vi "Config FTPSync.vi"(8 "error in (no error)":errorcluster, 11 "Cluster":T1) -> (0 "error out":errorcluster, 3 "FTPProtocol out":refnum<class "FTPProtocol.lvclass">)   [LabVIEW 2020, in "CSM-FileSync.lvlib" / "FTPProtocol.lvclass"]
uses:
  FTPProtocol.lvclass
  FTPProtocol.lvclass/FTPProtocol.ctl
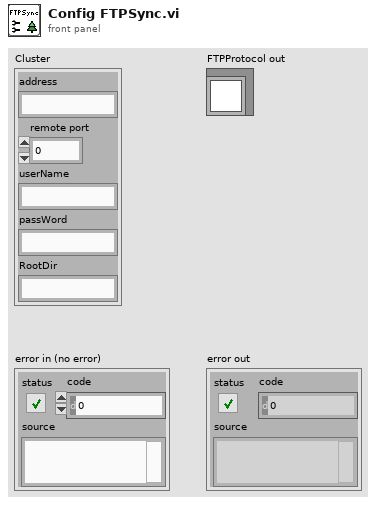
[diagram p1: front panel]
types:
  T1 = cluster{"address":string, "remote port":u16, "userName":string, "passWord":string, "RootDir":string}
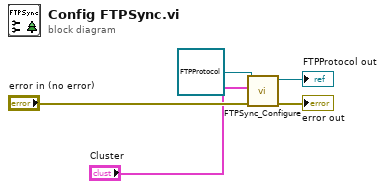
[diagram p0: block diagram]
diagram:
  n1 = call "FTPSync_Configure.vi"("error in (no error)"="error in (no error)", 10:"Cluster", "FTPProtocol in"=refnum<class "FTPProtocol.lvclass"> refnum ("FileSync -- FTP.lvlib:FTPProtocol")) -> ("error out"=→"error out":errorcluster, "FTPProtocol out"=→"FTPProtocol out":refnum<class "FTPProtocol.lvclass">)  [unwired: 7 in]
